vi "Cliente - Control.vi"() -> ()   [LabVIEW 2024]
uses:
  <vilib>/Analysis/2dsp.llb/Decimate (continuous, DBL).vi
  <vilib>/Analysis/NI_AALPro.lvlib
panel:
  out "Waveform Graph":dbl[](graph)
  in  "Tamaño ventana WL":i32=60
  in  "WL":dbl
  out "Waveform length":dbl[][](graph)
  out "number":u32
  in  "Limite superior WL":dbl=50.0
  in  "Limite inferior WL":dbl=25.0 format="%#_13g"
  in  "Escala autom. Y":u8=1
  in  "Maximo escala Y":dbl format="%#_13g"
  in  "Minimo escala Y":dbl format="%#_13g"
  in  "Minimo escala X":dbl
  in  "Maximo escala X":dbl
  in  "Escala autom. X":u8=1
  in  "Parar adquisicion 2":bool
  in  "factor decimacion":i32=20
  in  "tamaño buffer":i32=1000
  in  "Frecuencia muestreo":i32=20000
  in  "Server Closed":string="The server VI closed the connection."
  in  "Stop":bool
  out "*(type *) &x":dbl[](array[numeric])
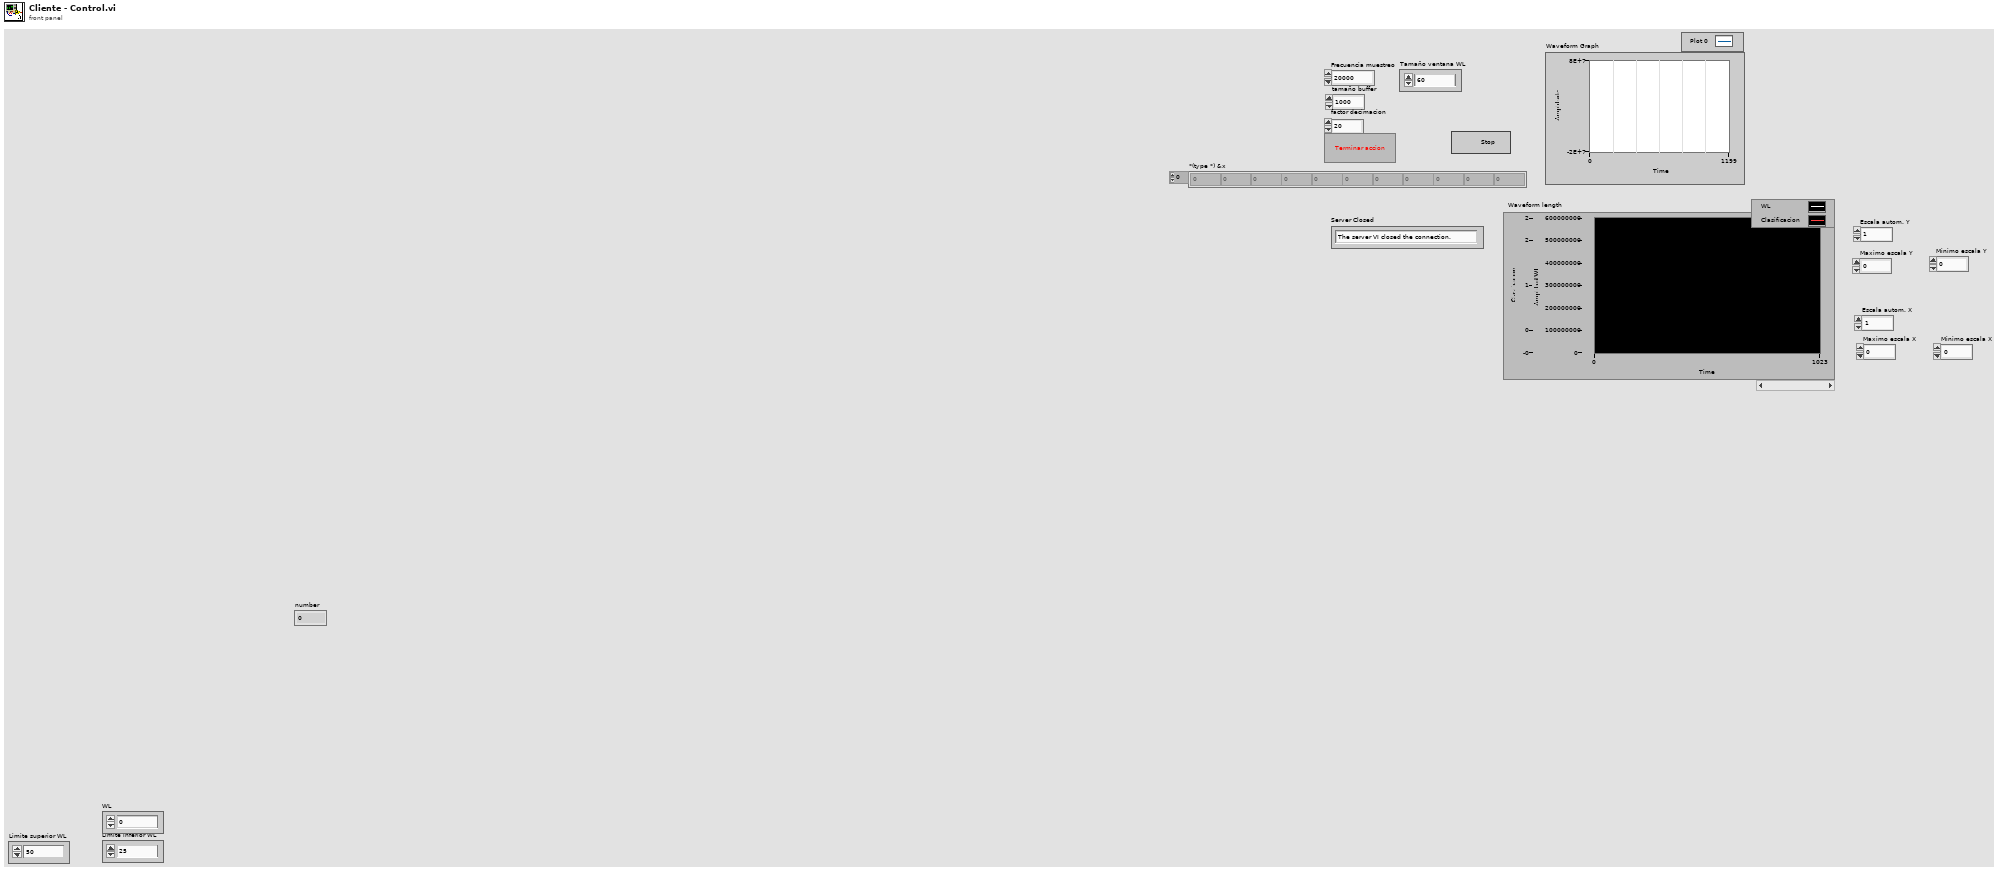
[diagram p1: front panel]
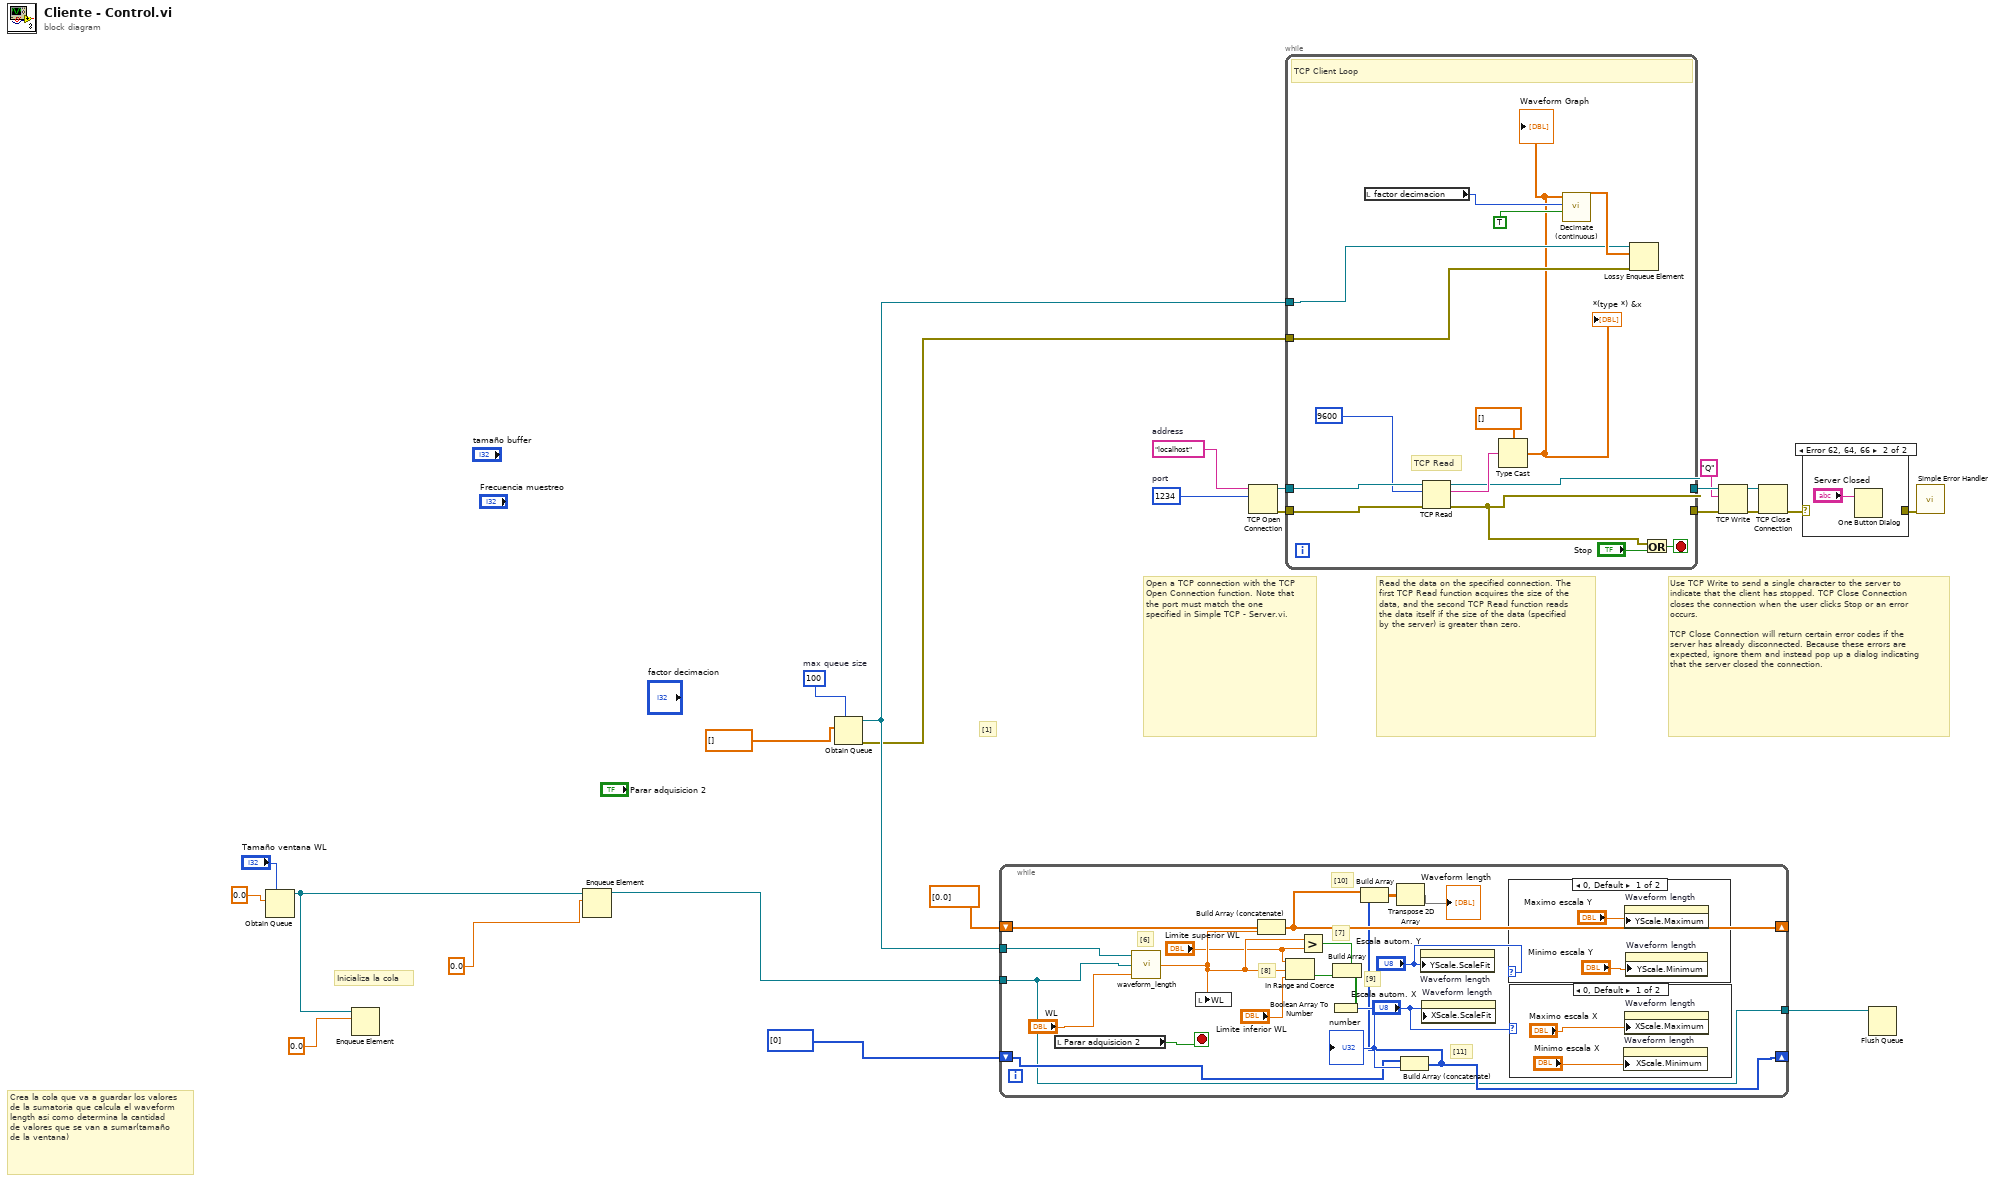
[diagram p0: block diagram]
diagram:
  w13 = 100  # max queue size
  w14 = u16 1234  # port
  w15 = "localhost"  # address
  # "Inicializa la cola"
  # "Crea la cola que va a guardar los valores de la sumatoria que calcula el waveform length así como determina la cantidad de valores que se van a sumar(tamaño de la ventana)"
  # "[1]"
  # "Use TCP Write to send a single character to the server to indicate that the client has stopped. TCP Close Connection closes the connection when the user clicks Stop or an error occurs.\n\nTCP Close Connection will return certain error codes if the server has already disconnected. Because these errors are expected, ignore them and instead pop up a dialog indicating that the server closed the connection."
  # "Read the data on the specified connection. The first TCP Read function acquires the size of the data, and the second TCP Read function reads the data itself if the size of the data (specified by the server) is greater than zero."
  # "Open a TCP connection with the TCP Open Connection function. Note that the port must match the one specified in Simple TCP - Server.vi."
  n1 = Obtain Queue(max queue size (-1, unlimited)="Tamaño ventana WL", element data type=0.0) -> (queue out=w3:refnum<queue>)  [unwired: 3 in, 2 out]
  n2 = Enqueue Element(queue=w3, element=0.0) -> ()  [unwired: 2 in, 3 out]
  n3 = Enqueue Element(queue=w3, element=0.0) -> (queue out=w9:refnum<queue>)  [unwired: 2 in, 2 out]
  n4 = Obtain Queue(max queue size (-1, unlimited)=w13, element data type=dbl[] [] ("Cola tipo")) -> (queue out=w2:refnum<queue>, error out=w1:errorcluster)  [unwired: 3 in, 1 out]
  n5 = while {
    tunnel: w9 -> [w26]
    tunnel: w2 -> [w43]
    shift-right: [w29] -> _
    shift-left: dbl[] [0.0] -> [w40]
    shift-right: [w28] -> _
    shift-left: u32[] [0] -> [w30]
    tunnel: [w26] -> w7
    stop <- w41 stop-if-true
    # "[11]"
    # "[10]"
    # "[9]"
    # "[8]"
    # "[7]"
    # "[6]"
    n6 = local read "Parar adquisicion 2"() -> (w41:bool)
    n7 = call "waveform_length.vi"("WL"="WL", "Cola WL"=w26, "Datos entrada"=w43) -> ("WL 2"=w38:dbl)
    n8 = local write "WL"(w38) -> ()
    n9 = Build Array (concatenate)(w40, w38) -> (w29:dbl[])
    n10 = In Range and Coerce(upper limit="Limite superior WL", x=w38, lower limit="Limite inferior WL") -> (In Range?=w36:bool)  [unwired: 1 out]
    n11 = Greater?(x=w38, y="Limite superior WL") -> (0:w37:bool)
    n12 = Build Array(w37, w36) -> (w35:bool[])
    n13 = Boolean Array To Number(Boolean array=w35) -> (number=w31:u32)
    "number" <- w31
    n14 = Build Array (concatenate)(w30, w31) -> (w28:u32[])
    n15 = Build Array(w29, w28) -> (w27:dbl[][])
    n16 = Transpose 2D Array(2D array=w27) -> (transposed array=→"Waveform length":dbl[][])
    n17 = property on="Waveform length" class="WFChart (strict)"("YScale.ScaleFit"="Escala autom. Y") -> ()  [unwired: 2 in, 2 out]
    n18 = property on="Waveform length" class="WFChart (strict)"("XScale.ScaleFit"="Escala autom. X") -> ()  [unwired: 2 in, 2 out]
    n19 = case shown="0, Default" "Escala autom. Y" {
      frame 0, Default {
        n20 = property on="Waveform length" class="WFChart (strict)"("YScale.Maximum"="Maximo escala Y") -> ()  [unwired: 2 in, 2 out]
        n21 = property on="Waveform length" class="WFChart (strict)"("YScale.Minimum"="Minimo escala Y") -> ()  [unwired: 2 in, 2 out]
      }
      frame 1 {
      }
    }
    n22 = case shown="0, Default" "Escala autom. X" {
      frame 0, Default {
        n23 = property on="Waveform length" class="WFChart (strict)"("XScale.Minimum"="Minimo escala X") -> ()  [unwired: 2 in, 2 out]
        n24 = property on="Waveform length" class="WFChart (strict)"("XScale.Maximum"="Maximo escala X") -> ()  [unwired: 2 in, 2 out]
      }
      frame 1 {
      }
    }
  }
  n25 = TCP Open Connection(address=w15, remote port or service name=w14) -> (connection ID=w24:refnum<k5>, error out=w23:errorcluster)  [unwired: 3 in]
  n26 = while {
    tunnel: w23 -> [w55]
    tunnel: w24 -> [w56]
    tunnel: [w57] -> w21
    tunnel: [w58] -> w19
    tunnel: w2 -> [w51]
    tunnel: w1 -> [w50]
    stop <- w61 stop-if-true
    # "TCP Read"
    # "TCP Client Loop"
    n27 = local read "factor decimacion"() -> (w52:i32)
    n28 = TCP Read(connection ID=w56, bytes to read=9600, error in (no error)=w55) -> (connection ID out=w57:refnum<k5>, data out=w60:string, error out=w58:errorcluster)  [unwired: 2 in]
    n29 = Type Cast(type=dbl[] [] ("chart"), x=w60) -> (*(type *) &x=w48:dbl[])
    "*(type *) &x" <- w48
    "Waveform Graph" <- w48
    n30 = call-poly <vilib>:"Decimate (continuous).vi"("averaging"=TRUE, "decimating factor"=w52, "X"=w48) -> ("Decimated Array"=w53:dbl[])  [unwired: 7 in, 1 out]
    n31 = Lossy Enqueue Element(queue=w51, element=w53, error in (no error)=w50) -> ()  [unwired: 4 out]
    n32 = Or(x=w58, y="Stop") -> (x .or. y?=w61:bool)
  }
  n33 = TCP Write(connection ID=w21, data in="Q", error in (no error)=w19) -> (connection ID out=w22:refnum<k5>, error out=w20:errorcluster)  [unwired: 2 out]
  n34 = TCP Close Connection(connection ID=w22, error in (no error)=w20) -> (error out=w17:errorcluster)  [unwired: 1 in, 1 out]
  n35 = case shown="Error 62, 64, 66" w17 {
    selector: w17 -> [w63 _]
    tunnel: [w63 _] -> w16
    frame #0 {
    }
    frame #1 {
      n36 = One Button Dialog(message="Server Closed") -> ()  [unwired: 1 in, 1 out]
    }
  }
  n37 = Flush Queue(queue=w7) -> ()  [unwired: 1 in, 3 out]
  n38 = call <vilib>:"Simple Error Handler.vi"("error in (no error)"=w16) -> ()  [unwired: 4 in, 5 out]
